vi "Dialog_AppendLayout(s).vi"(4 "Viewer Layout Ref":refnum<vi>, 5 "SetList Layout Ref":refnum<vi>, 6 "View Col array":refnum<class "Column.lvclass">[](array[class]), 7 "Col Array Refnum":refnum<vi>, 10 "SetList DevNums":i32[](array[numeric]), 11 "SetList Dev queue":refnum<queue>) -> ()   [LabVIEW 2013]
uses:
  DeviceVIs/Device/Device.lvclass
  ColumnVIs/Column/Column.lvclass
  <vilib>/Utility/miscctls.llb/LVStringsAndValuesArrayTypeDef_I32.ctl
panel:
  in  "Cancel":bool
  in  "OK":bool
  in  "Listbox":i32(listbox) caption="Click to select layouts to import:"
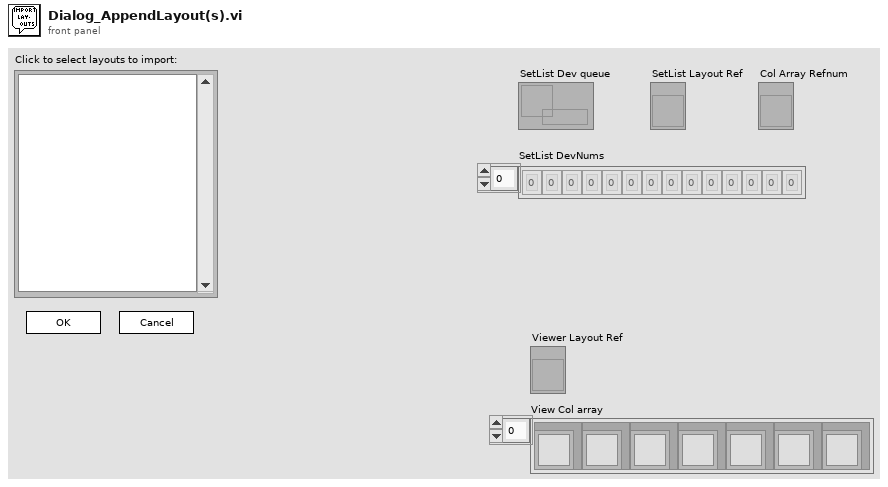
[diagram p1: front panel]
types:
  T1 = typedef "LVStringsAndValuesArrayTypeDef_I32.ctl" = cluster{"String":string, "Value":i32}[]
  T2 = typedef "ColumnLayoutCluster.ctl" = cluster{"Label":string, "Color":u32, "Width":u32, "[disp?]":bool[]}
  T3 = typedef "LVPoint32TypeDef.ctl" = cluster{"Horizontal":i32, "Vertical":i32}
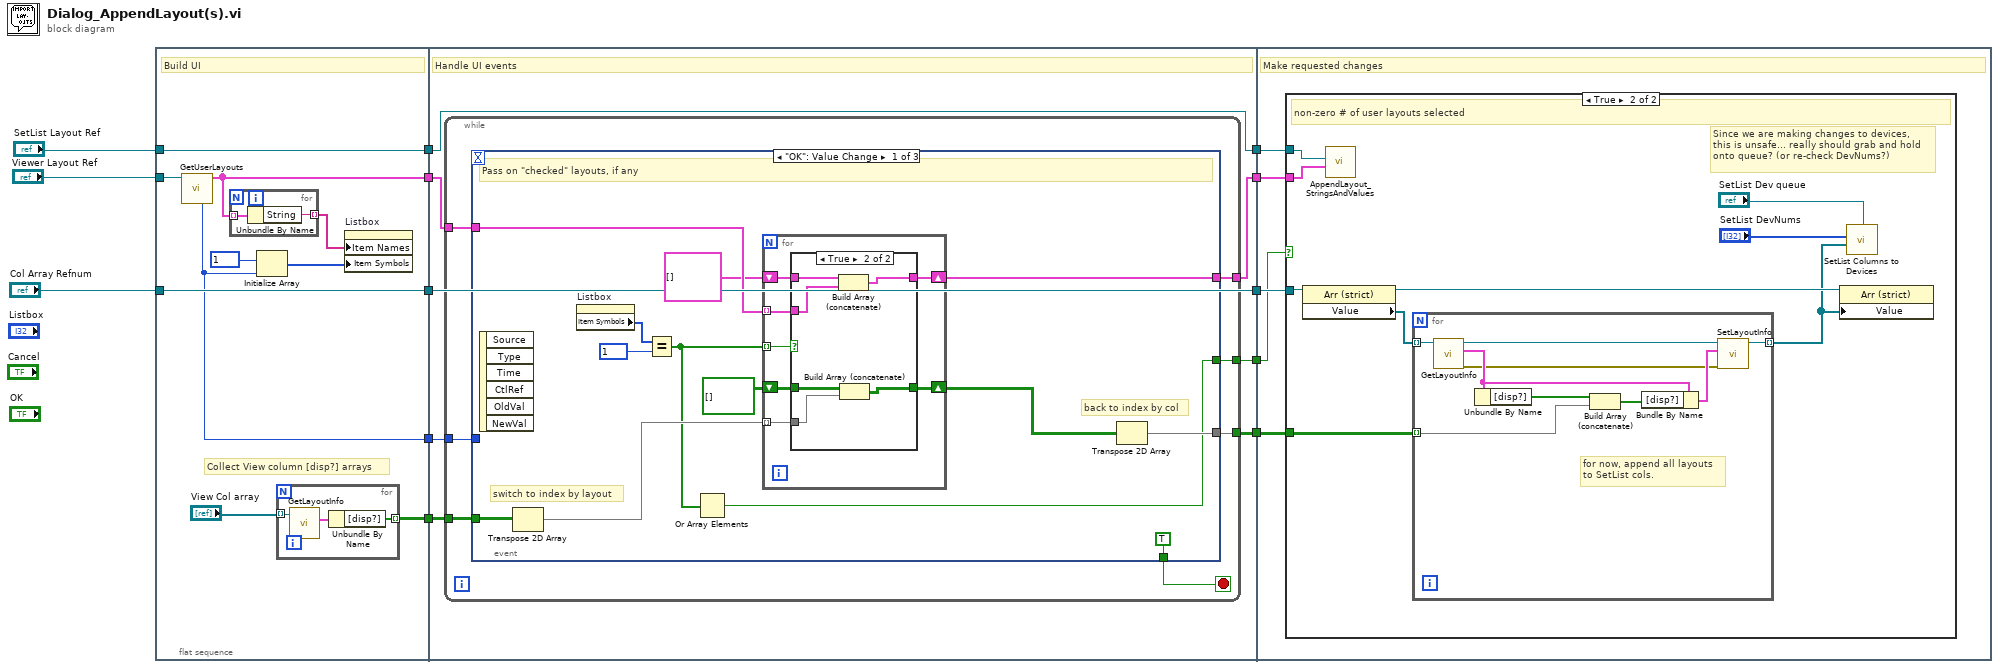
[diagram p0: block diagram]
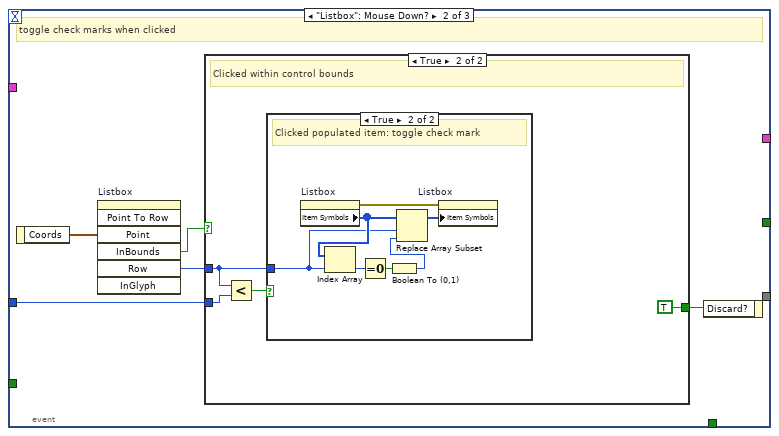
[diagram p3: hidden frame]
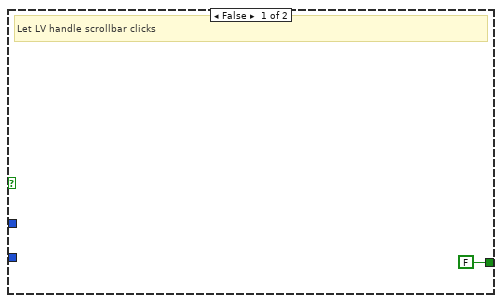
[diagram p4: hidden frame]
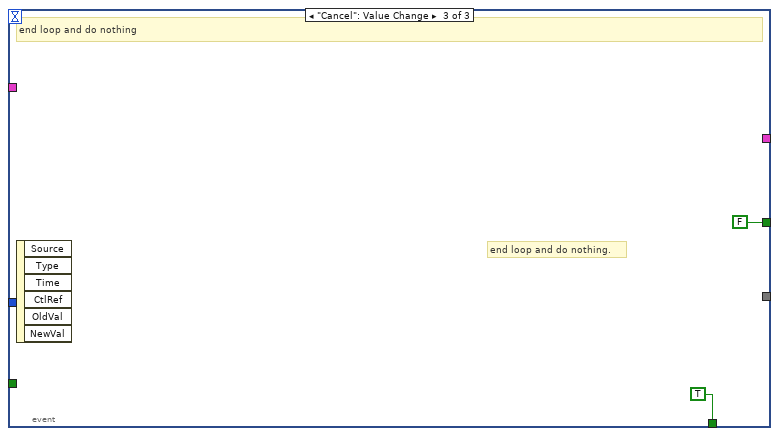
[diagram p6: hidden frame]
diagram:
  n1 = flat-sequence {
    tunnel: "Col Array Refnum" -> [w22]
    tunnel: "SetList Layout Ref" -> [w23]
    tunnel: [w18] -> w8
    tunnel: [w23] -> w7
    tunnel: [w22] -> w6
    tunnel: "Viewer Layout Ref" -> [w21]
    tunnel: [w16] -> w3
    tunnel: [w14] -> w2
    tunnel: [w29] -> w11
    tunnel: [w36] -> w10
    tunnel: [w35] -> w9
    tunnel: w8 -> [w32]
    tunnel: w7 -> [w36]
    tunnel: w6 -> [w35]
    tunnel: [w34] -> w4
    tunnel: w3 -> [w33]
    tunnel: w2 -> [w31]
    tunnel: [w30] -> w1
    tunnel: w11 -> [w95]
    tunnel: w10 -> [w94]
    tunnel: w9 -> [w93]
    tunnel: w4 -> [w92]
    tunnel: w1 -> [w91]
    frame #0 {
      # "Collect View column [disp?] arrays"
      # "Build UI"
      n2 = call "GetUserLayouts.vi"("Layout Ring Refnum"=w21) -> ("User StringsAndValues[]"=w18:T1, "Num User Layouts"=w16:i32)  [unwired: 6 in, 3 out]
      n3 = for {
        tunnel: w18 -> [w28] mode=indexing
        tunnel: [w27] -> w17 mode=indexing
        n4 = Unbundle By Name(w28) -> ("String"=w27:string)
      }
      n5 = Initialize Array(1, w16) -> (w19:i32[])
      n6 = for {
        tunnel: "View Col array" -> [w25] mode=indexing
        tunnel: [w24] -> w14 mode=indexing
        n7 = call "GetLayoutInfo.vi"("Column in"=w25) -> ("Layout cluster"=w26:T2)  [unwired: 8 in, 2 out]
        n8 = Unbundle By Name(w26) -> ("[disp?]"=w24:bool[])
      }
      n9 = property on="Listbox" class="LstBox (strict)"("Item Names"=w17, "Item Symbols"=w19) -> ()  [unwired: 2 in, 2 out]
    }
    frame #1 {
      # "Handle UI events"
      n10 = while {
        tunnel: [w42] -> w34
        tunnel: w33 -> [w41]
        tunnel: w32 -> [w40]
        tunnel: w31 -> [w39]
        tunnel: [w38] -> w30
        tunnel: [w37] -> w29
        stop <- w43 stop-if-true
        n11 = event shown="[0] \"OK\": Value Change" {
          selector: _ -> [_ _ _]
          dyn-events: _ -> [_ _ _]
          timeout: _ -> [_ _ _]
          tunnel: [TRUE _ TRUE] -> w43
          tunnel: [w45 _ FALSE] -> w42
          tunnel: w41 -> [_ w72 _]
          tunnel: w40 -> [w53 _ _]
          tunnel: w39 -> [w52 _ _]
          tunnel: [w47 _ _] -> w38
          tunnel: [w44 _ _] -> w37
          event "OK": Value Change {
            # "back to index by col"
            # "switch to index by layout"
            # "Pass on \"checked\" layouts, if any"
            n12 = event-data() -> ()  [unwired: 1 in, 6 out]
            n13 = Transpose 2D Array(2D array=w52) -> (transposed array=w51:bool[][])
            n14 = property on="Listbox" class="LstBox (strict)"() -> ("Item Symbols"=w55:i32[])  [unwired: 2 in, 2 out]
            n15 = Equal?(x=w55, y=1) -> (x = y?=w46:bool[])
            n16 = Or Array Elements(Boolean array=w46) -> (logical OR=w45:bool)
            n17 = for {
              tunnel: w53 -> [w58] mode=indexing
              tunnel: w46 -> [w63] mode=indexing
              tunnel: w51 -> [w57] mode=indexing
              shift-right: [w61] -> w44
              shift-left: T1 [] ("User StringsAndValues[]") -> [w62]
              shift-right: [w59] -> w48
              shift-left: bool[][] [] ("transposed array") -> [w60]
              n18 = case shown="True" w63 {
                tunnel: w62 -> [w65 w71]
                tunnel: [w65 w69] -> w61
                tunnel: w60 -> [w64 w68]
                tunnel: [w64 w66] -> w59
                tunnel: w58 -> [_ w70]
                tunnel: w57 -> [_ w67]
                frame False {
                }
                frame True {
                  n19 = Build Array (concatenate)(w71, w70) -> (w69:T1)
                  n20 = Build Array (concatenate)(w68, w67) -> (w66:bool[][])
                }
              }
            }
            n21 = Transpose 2D Array(2D array=w48) -> (transposed array=w47:bool[][])
          }
          event "Listbox": Mouse Down? {
            # "toggle check marks when clicked"
            n22 = event-data() -> ("Coords"=w76:T3)  [unwired: 1 in]
            n23 = invoke on="Listbox" class="LstBox (strict)" method="Point To Row"("Point"=w76) -> ("InBounds"=w74:bool, "Row"=w75:i32)  [unwired: 6 in, 5 out]
            n24 = case shown="True" w74 {
              tunnel: w75 -> [_ w79]
              tunnel: [FALSE TRUE] -> w73
              tunnel: w72 -> [_ w80]
              frame False {
                # "Let LV handle scrollbar clicks"
              }
              frame True {
                # "Clicked within control bounds"
                n25 = Less?(x=w79, y=w80) -> (x < y?=w78:bool)
                n26 = case shown="True" w78 {
                  tunnel: w79 -> [_ w82]
                  frame False {
                    # "clicked below populated items: do nothing"
                  }
                  frame True {
                    # "Clicked populated item: toggle check mark"
                    n27 = property on="Listbox" class="LstBox (strict)"() -> (error out=w83:errorcluster, "Item Symbols"=w85:i32[])  [unwired: 2 in, 1 out]
                    n28 = Index Array(array=w85, index=w82) -> (element=w86:i32)
                    n29 = Equal To 0?(x=w86) -> (x = 0?=w88:bool)
                    n30 = Boolean To (0,1)(Boolean=w88) -> (0, 1=w87:i16)
                    n31 = Replace Array Subset(array=w85, new element=w87, index=w82) -> (w84:i32[])
                    n32 = property on="Listbox" class="LstBox (strict)"(error in=w83, "Item Symbols"=w84) -> ()  [unwired: 1 in, 2 out]
                  }
                }
              }
            }
            n33 = event-data("Discard?"=w73) -> ()  [unwired: 1 in, 1 out]
          }
          event "Cancel": Value Change {
            # "end loop and do nothing."
            # "end loop and do nothing"
            n34 = event-data() -> ()  [unwired: 1 in, 6 out]
          }
        }
      }
    }
    frame #2 {
      # "Make requested changes"
      n35 = case shown="True" w92 {
        tunnel: w95 -> [_ w101]
        tunnel: w94 -> [_ w102]
        tunnel: w93 -> [_ w100]
        tunnel: w91 -> [_ w96]
        frame False {
          # "no layouts to add!"
        }
        frame True {
          # "Since we are making changes to devices,\nthis is unsafe... really should grab and hold\nonto queue? (or re-check DevNums?)"
          # "non-zero # of user layouts selected"
          n36 = property class="Arr (strict)"(reference=w100) -> (reference out=w98:refnum<vi>, "Value"=w99:refnum<class "Column.lvclass">[])  [unwired: 1 in, 1 out]
          n37 = call "AppendLayout_StringsAndValues.vi"("StringsAndValues[] to apend"=w101, "SetList Layout Ref"=w102) -> ()  [unwired: 10 in]
          n38 = for {
            tunnel: w99 -> [w113] mode=indexing
            tunnel: [w106] -> w97 mode=indexing
            tunnel: w96 -> [w105] mode=indexing
            # "for now, append all layouts\nto SetList cols."
            n39 = call "GetLayoutInfo.vi"("Column in"=w113) -> ("error out"=w107:errorcluster, "Layout cluster"=w110:T2, "Column out"=w112:refnum<class "Column.lvclass">)  [unwired: 8 in]
            n40 = Unbundle By Name(w110) -> ("[disp?]"=w111:bool[])
            n41 = Build Array (concatenate)(w111, w105) -> (w109:bool[])
            n42 = Bundle By Name(cluster=w110, "[disp?]"=w109) -> (w108:T2)
            n43 = call "SetLayoutInfo.vi"("error in (no error)"=w107, "Layout cluster"=w108, "Column in"=w112) -> ("Column out"=w106:refnum<class "Column.lvclass">)  [unwired: 7 in, 1 out]
          }
          n44 = property class="Arr (strict)"(reference=w98, "Value"=w97) -> ()  [unwired: 1 in, 2 out]
          n45 = call "SetList Columns to Devices.vi"("Col array in"=w97, "DevNums In"="SetList DevNums", "Devices queue"="SetList Dev queue") -> ()  [unwired: 7 in, 2 out]
        }
      }
    }
  }
